vi "labviewww tania 3.vi"() -> ()   [LabVIEW 2011]
panel:
  out "Contador":dbl
  out "Menor":dbl
  out "Mayor":dbl
  out "Promedio":dbl
  out "Temperatura":dbl(slide) scale=0.0..100.0
  # "Generar 10 temperaturas y al final presentar la temperatura mayor, menor y la temperatura promedio."
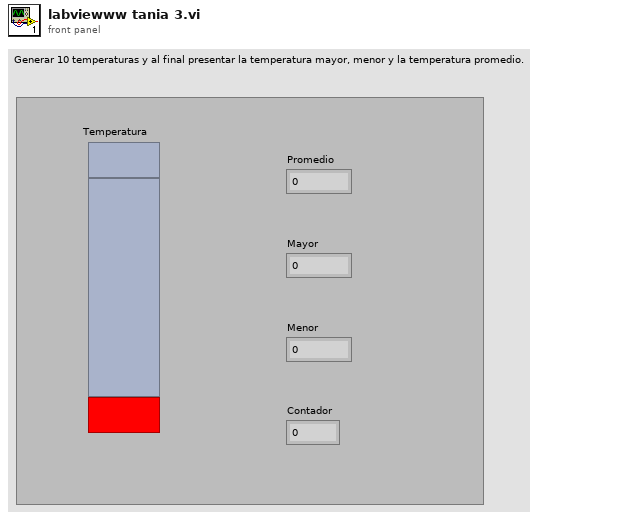
[diagram p1: front panel]
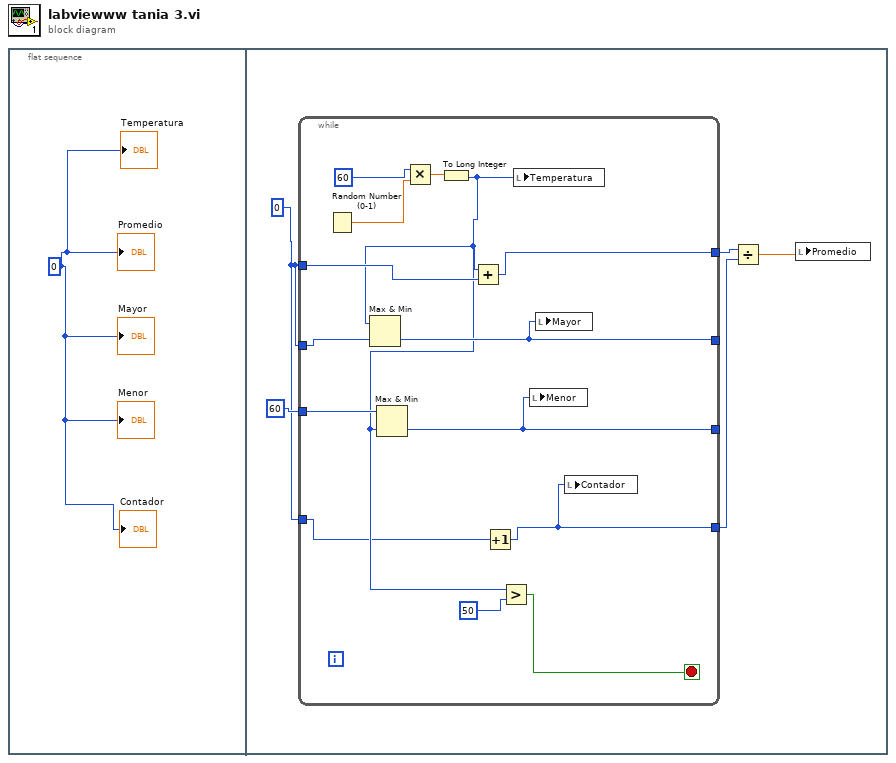
[diagram p0: block diagram]
diagram:
  n1 = flat-sequence {
    frame #0 {
      w1 = 0
      "Temperatura" <- w1
      "Promedio" <- w1
      "Mayor" <- w1
      "Menor" <- w1
      "Contador" <- w1
    }
    frame #1 {
      w3 = 0
      n2 = while {
        tunnel: w3 -> [w17]
        tunnel: [w16] -> w6
        tunnel: w3 -> [w15]
        tunnel: 60 -> [w14]
        tunnel: [w12] -> _
        tunnel: [w13] -> _
        tunnel: w3 -> [w8]
        tunnel: [w7] -> w2
        stop <- w9 stop-if-true
        n3 = Random Number (0-1)() -> (number: 0 to 1=w19:dbl)
        n4 = Multiply(x=60, y=w19) -> (x*y=w18:dbl)
        n5 = To Long Integer(number=w18) -> (32bit integer=w10:i32)
        n6 = Max & Min(x=w10, y=w15) -> (min(x,y)=w13:i32)  [unwired: 1 out]
        n7 = Max & Min(x=w14, y=w10) -> (min(x,y)=w12:i32)  [unwired: 1 out]
        n8 = Add(x=w10, y=w17) -> (x+y=w16:i32)
        n9 = Increment(x=w8) -> (x+1=w7:i32)
        n10 = Greater?(x=w10, y=50) -> (0:w9:bool)
        n11 = local write "Temperatura"(w10) -> ()
        n12 = local write "Menor"(w12) -> ()
        n13 = local write "Mayor"(w13) -> ()
        n14 = local write "Contador"(w7) -> ()
      }
      n15 = Divide(x=w6, y=w2) -> (x/y=w5:dbl)
      n16 = local write "Promedio"(w5) -> ()
    }
  }
